vi "ISX3_Cmd_SetSetupCalibrationInteraction.vi"(1 "Calibration Value":sgl, 2 "Load Type":u8(ring)=1 items=["Resistance"=1, "Capacitator"=2]) -> (0 "set Setup Start Calibration Cmd":u8[](array[numeric]))   [LabVIEW 2012, in "Sciospec ISX3 Impedance Analyzer.lvlib"]
uses:
  Sciospec ISX3 Impedance Analyzer.lvlib
panel:
  # "This VI generates the command to answer the calibration interaction.\nDepending on the calibration case the \"Load Type\" determine if the \ncalibration load object is a capacitor or a resistor.\nDepending on  the \"Load Type\" the calibration value is in Farad or in Ohm."
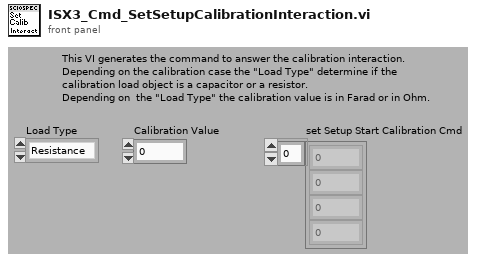
[diagram p1: front panel]
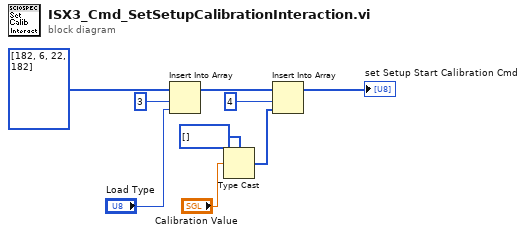
[diagram p0: block diagram]
diagram:
  n1 = Insert Into Array(array=u8[] [182, 6, 22, 182], index=3, new element="Load Type") -> (w6:u8[])
  n2 = Type Cast(type=u8[] [], x="Calibration Value") -> (*(type *) &x=w3:u8[])
  n3 = Insert Into Array(array=w6, index=4, new element=w3) -> (→"set Setup Start Calibration Cmd":u8[])
